vi "Main_001.vi"() -> ()   [LabVIEW 2018]
uses:
  Control/State_01.ctl
  <vilib>/vision/Image Controls.llb/IMAQ Image.ctl
  <vilib>/Utility/miscctls.llb/LVRectTypeDef.ctl
  <vilib>/Utility/miscctls.llb/LVPointTypeDef.ctl
  <vilib>/Utility/file.llb/Write Delimited Spreadsheet (string).vi
  <vilib>/vision/NI_Vision_Development_Module.lvlib
panel:
  out "OCR":bool
  out "Batch":bool
  in  "BatchCycle_Control":u32
  out "BatchCycle":u32
  out "stripped path":path
  in  "Type of Symmetry 4":u32(ring) items=["Horizontal", "Vertical", "Central", "1st Diagonal", "2nd Diagonal"]
  in  "Type of Symmetry":u32(ring)=1 items=["Horizontal", "Vertical", "Central", "1st Diagonal", "2nd Diagonal"]
  in  "Type of Symmetry 3":u32(ring)=1 items=["Horizontal", "Vertical", "Central", "1st Diagonal", "2nd Diagonal"]
  in  "Type of Symmetry 2":u32(ring)=2 items=["Horizontal", "Vertical", "Central", "1st Diagonal", "2nd Diagonal"]
  in  "TrainFile Path":path=path "D:/Life/20191001_Accordance/Project/EPISIL/20200806-Camera/LabVIEW_Test/OCR"
  in  "error in (no error)":errorcluster
  out "error out":errorcluster
  in  "Button_Batch":bool
  in  "Button_EXIT":bool
  out "Result_04":string
  out "Result_03":string
  out "Result_02":string
  out "Result_01":string
  in  "Button_OCR":bool
  in  "Button_ROI":bool
  in  "Erode_04":i32
  in  "Dilate_04":i32
  in  "Y+H_04":i32=990
  in  "X_04":i32=1330
  in  "Y_04":i32=1050
  in  "X+W_04":i32=1390
  out "Show_04":T1(plugin-control)
  in  "Erode_03":i32
  in  "Dilate_03":i32
  in  "Y+H_03":i32=890
  in  "X_03":i32=1380
  in  "Y_03":i32=960
  in  "X+W_03":i32=1450
  out "Show_03":T1(plugin-control)
  in  "Erode_02":i32
  in  "Dilate_02":i32
  in  "Y+H_02":i32=1000
  in  "X_02":i32=650
  in  "Y_02":i32=910
  in  "X+W_02":i32=870
  out "Show_02":T1(plugin-control)
  in  "Binary Value":i32
  in  "Erode_01":i32
  in  "Dilate_01":i32
  in  "Y+H_01":i32=400
  in  "X_01":i32=685
  in  "Y_01":i32=300
  in  "X+W_01":i32=885
  in  "ImagePath":path=path "D:/Life/20191001_Accordance/Project/EPISIL/20200806-Camera/20200716/getimg_003.bmp"
  out "Show_01":T1(plugin-control)
  # "X"
  # "Y"
  # "X+W"
  # "Y+H"
  # "Dilate"
  # "Erode"
  # "X"
  # "Y"
  # "X+W"
  # "Y+H"
  # "Dilate"
  # "Erode"
  # "X"
  # "Y"
  # "X+W"
  # "Y+H"
  # "Dilate"
  # "Erode"
  # "X"
  # "Y"
  # "X+W"
  # "Y+H"
  # "Dilate"
  # "Erode"
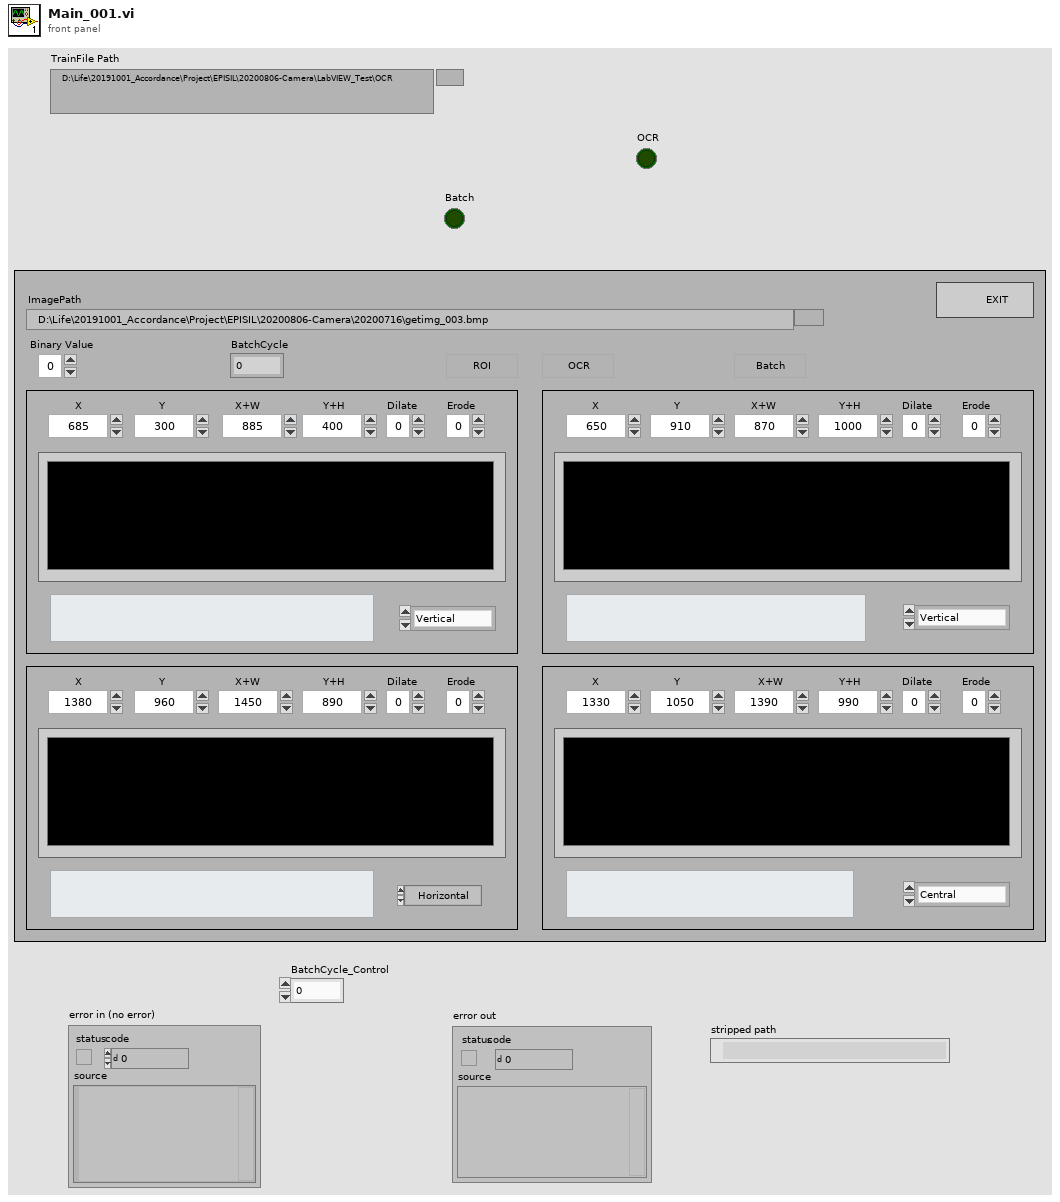
[diagram p1: front panel]
types:
  T1 = typedef "IMAQ Image.ctl" = refnum<image>
  T2 = typedef "State_01.ctl" = enum16{"Inital", "Disable", "Idle", "Display", "BatchCompare", "ROI_01", "ROI_02", "ROI_03", "ROI_04", "OCR", "SaveResult", "EXIT"}
  T3 = typedef "IMAQ OCR Session.ctl" = refnum<k1>
  T4 = typedef "LVPointTypeDef.ctl" = cluster{"Horizontal":i16, "Vertical":i16}
  T5 = typedef "LVRectTypeDef.ctl" = cluster{"Left":i16, "Top":i16, "Right":i16, "Bottom":i16}
  T6 = typedef "IMAQ Rectangle" = cluster{"Left":i32, "Top":i32, "Right":i32, "Bottom":i32, "Rotation":dbl}
  T7 = typedef "Image Type" = u32
  T8 = typedef "ROI Descriptor" = cluster{"Global Rectangle":i32[], "Contours":cluster{"ID":enum32{"External", "Internal"}, "Type":u32, "Coordinates":i32[]}[]}
  T9 = cluster{"Global Rectangle":i32[], "Contours":cluster{"ID":enum32{"External", "Internal"}, "Type":u32, "Coordinates":i32[]}[]}
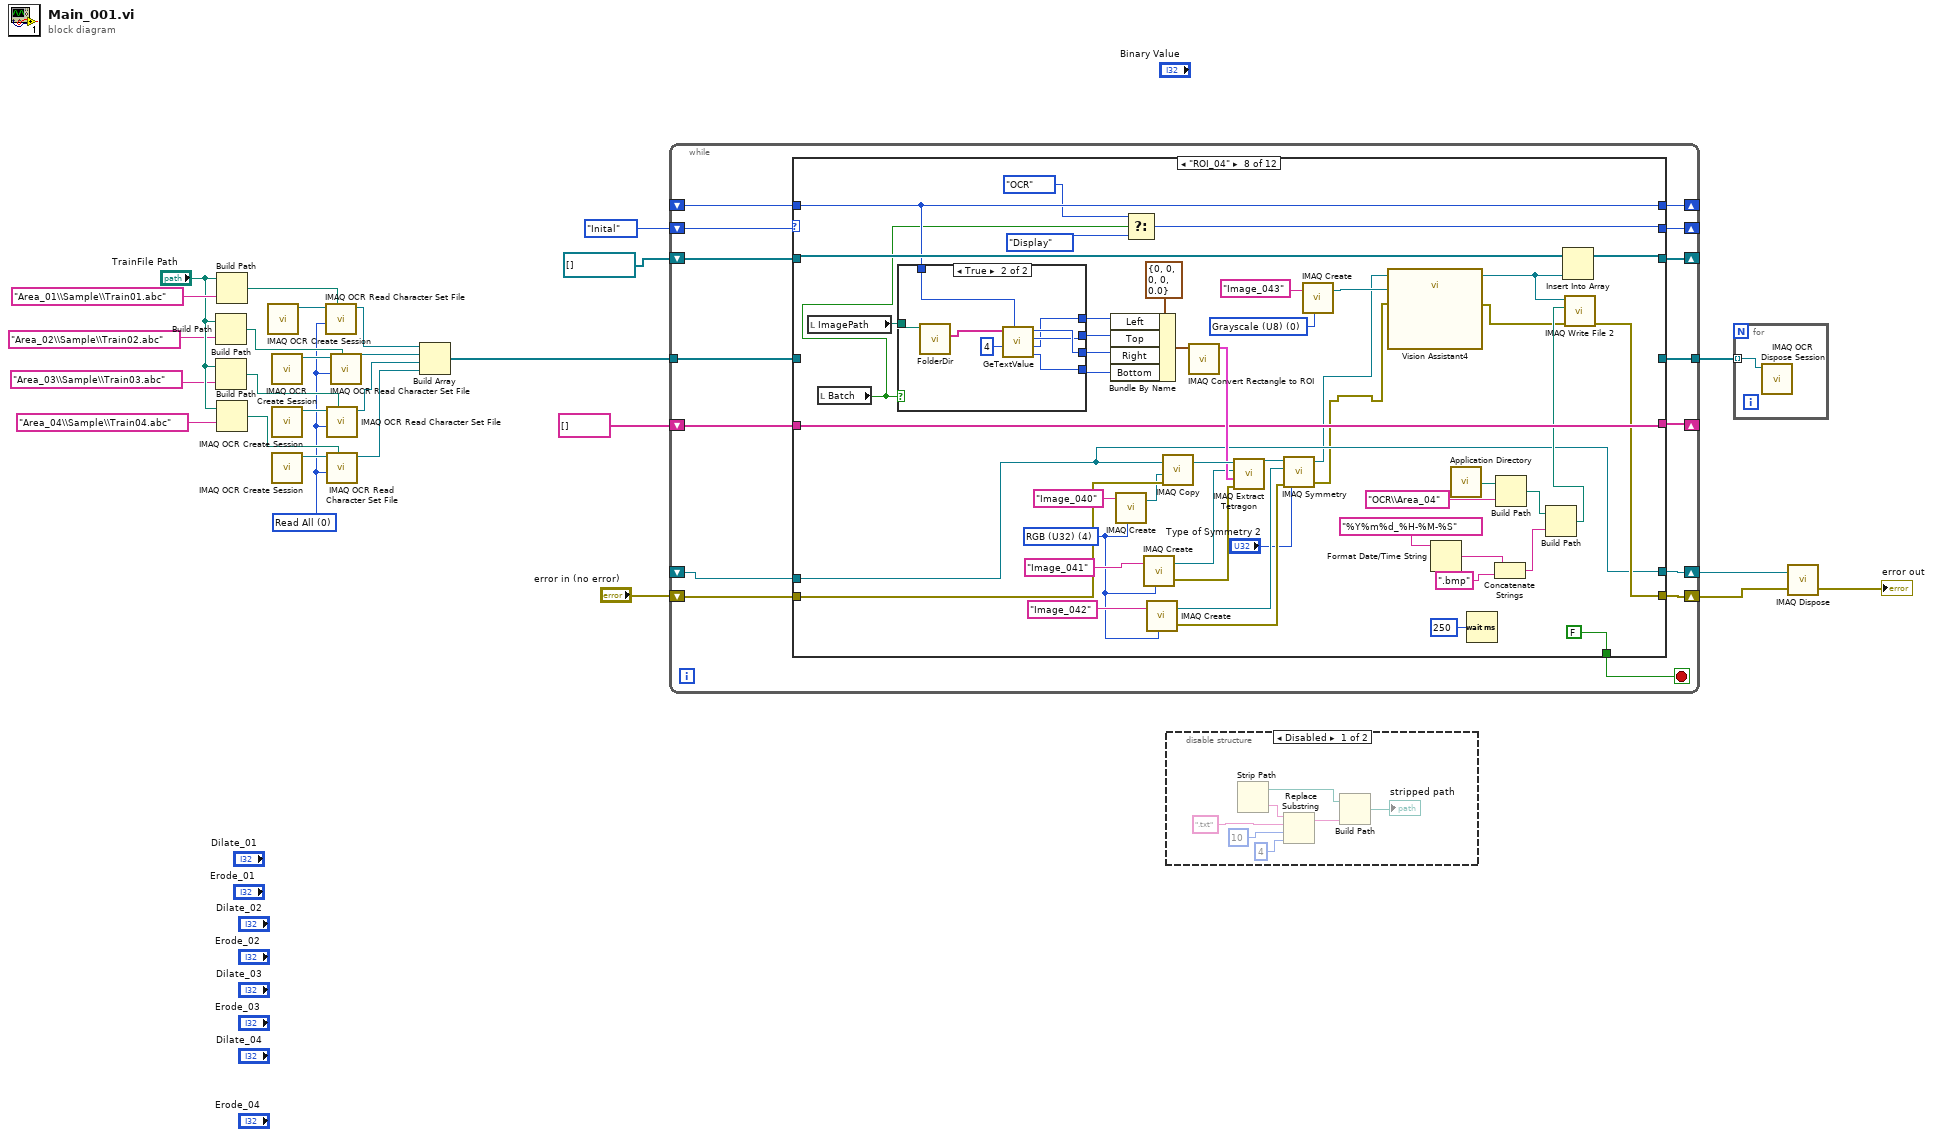
[diagram p0: block diagram]
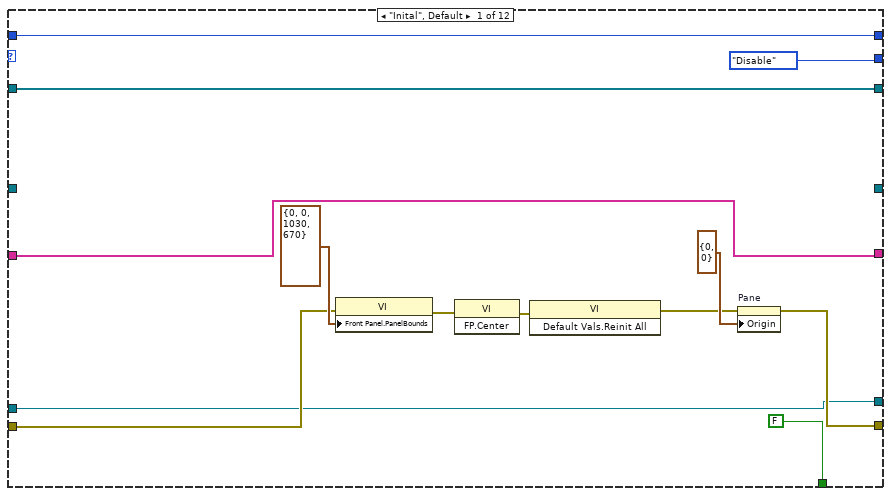
[diagram p3: hidden frame]
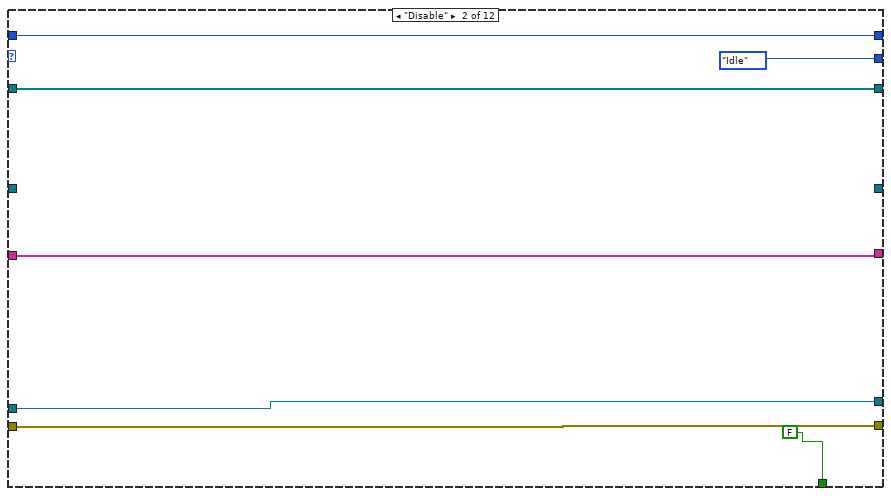
[diagram p4: hidden frame]
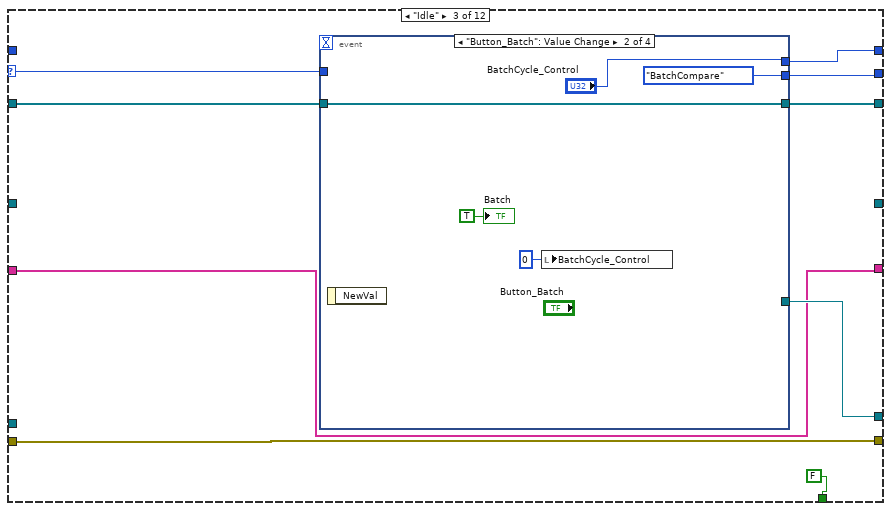
[diagram p5: hidden frame]
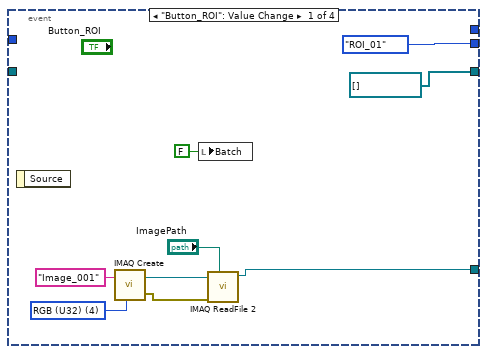
[diagram p6: hidden frame]
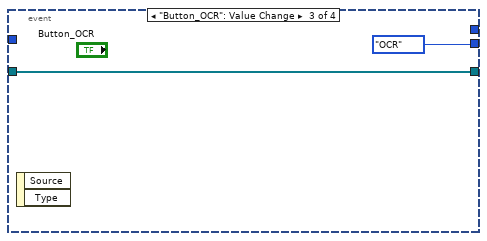
[diagram p7: hidden frame]
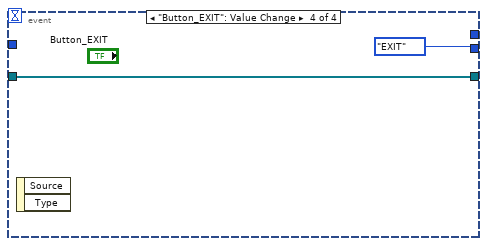
[diagram p8: hidden frame]
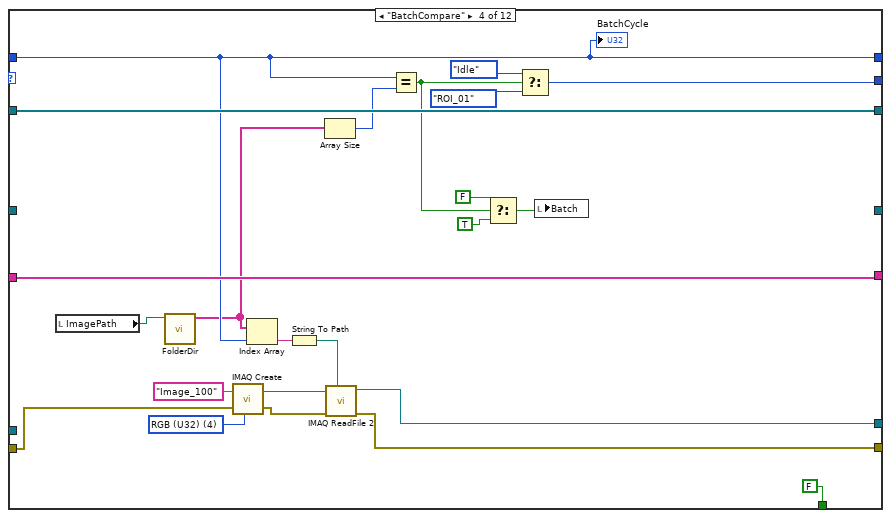
[diagram p9: hidden frame]
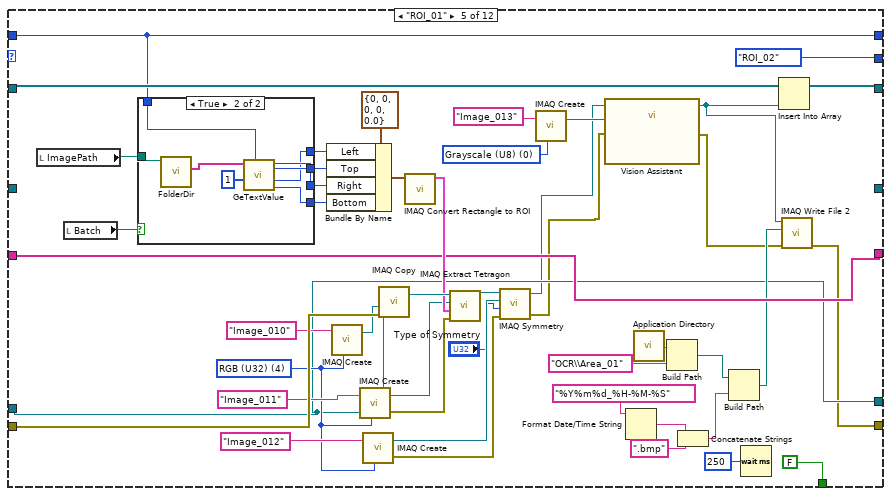
[diagram p10: hidden frame]
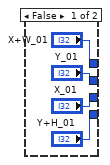
[diagram p11: hidden frame]
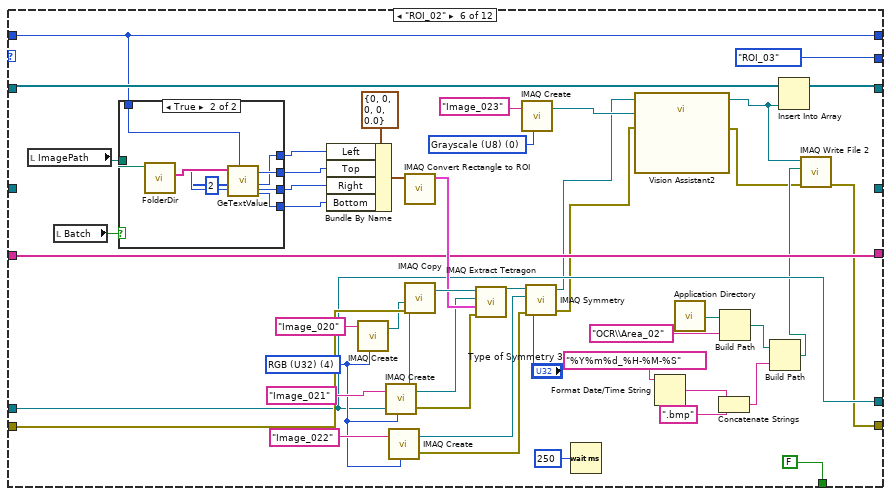
[diagram p12: hidden frame]
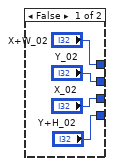
[diagram p13: hidden frame]
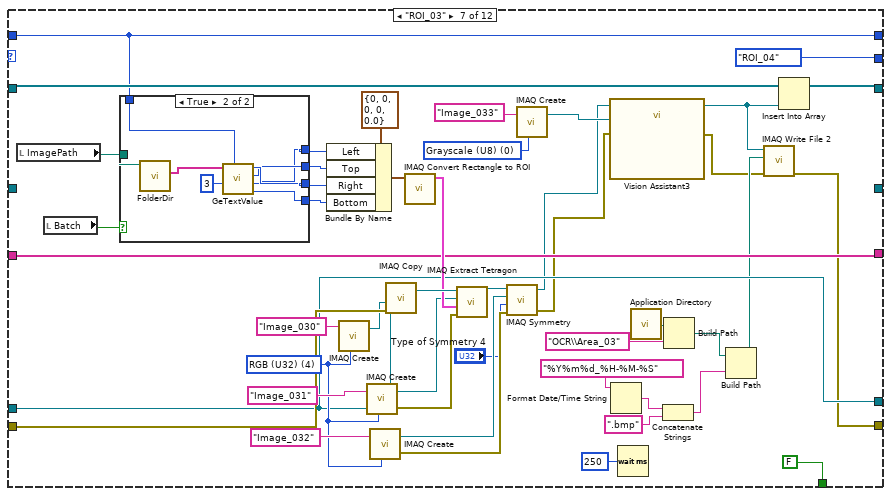
[diagram p14: hidden frame]
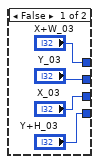
[diagram p15: hidden frame]
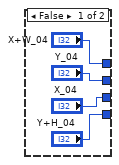
[diagram p16: hidden frame]
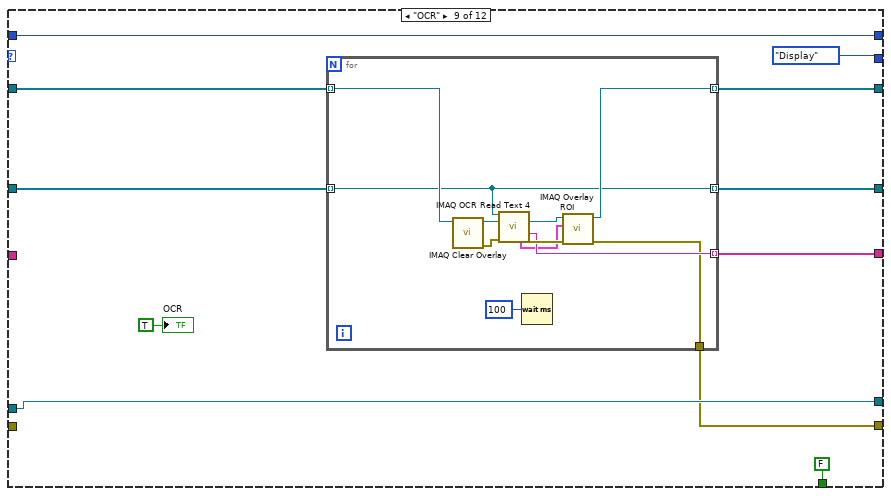
[diagram p17: hidden frame]
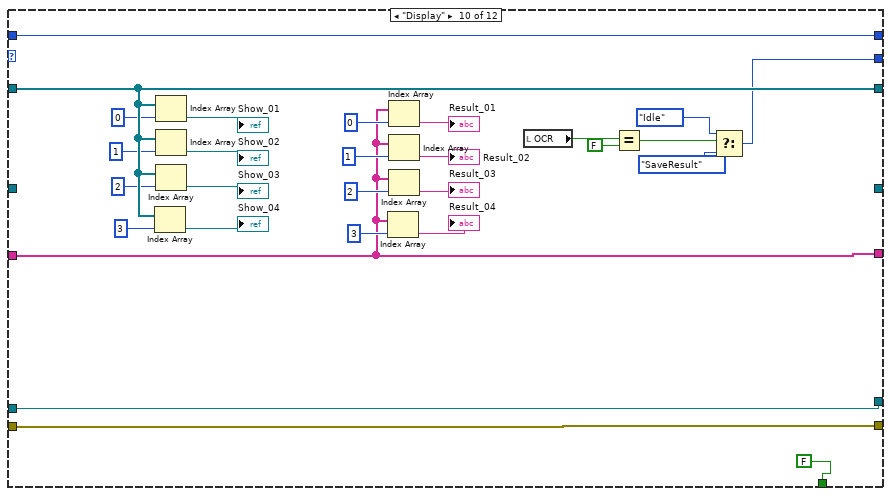
[diagram p18: hidden frame]
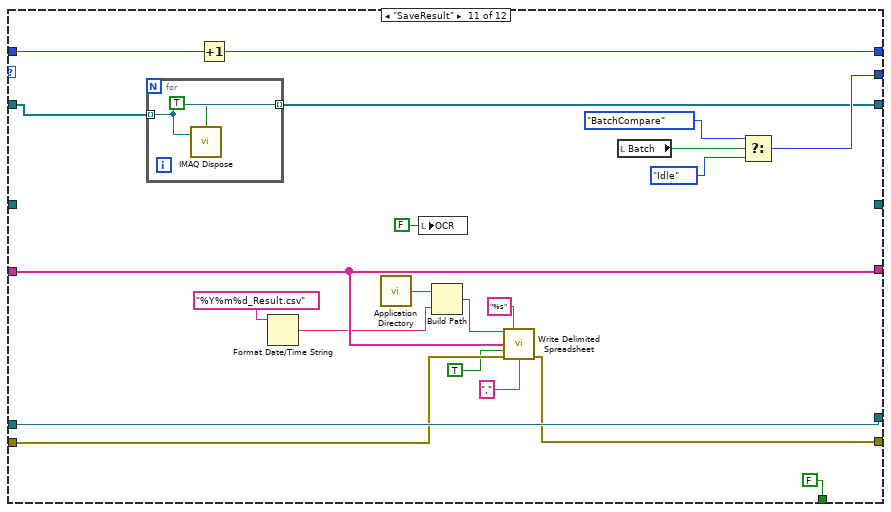
[diagram p19: hidden frame]
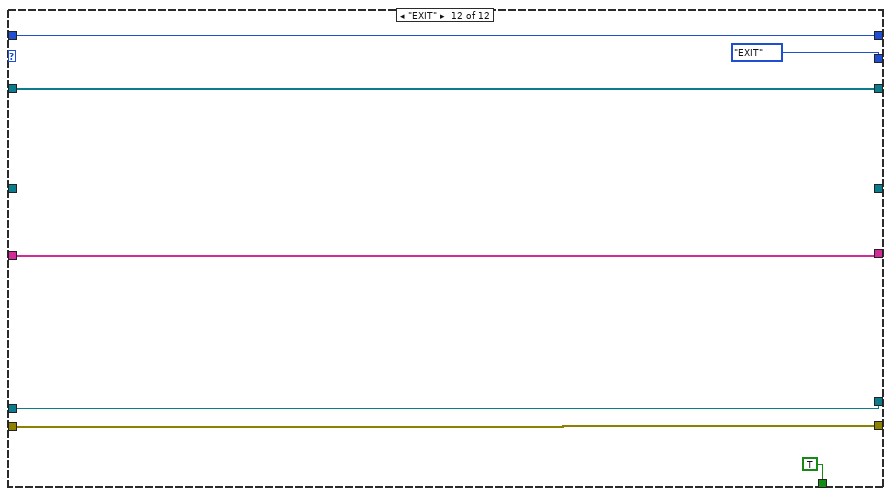
[diagram p20: hidden frame]
diagram:
  w7 = 0 items=["Read All", "Read Character Set Only", "Read Properties Only"] ("Read Options")
  n1 = Build Path(base path="TrainFile Path", name or relative path="Area_02\\Sample\\Train02.abc") -> (appended path=w12:path)
  n2 = Build Path(base path="TrainFile Path", name or relative path="Area_03\\Sample\\Train03.abc") -> (appended path=w11:path)
  n3 = Build Path(base path="TrainFile Path", name or relative path="Area_01\\Sample\\Train01.abc") -> (appended path=w15:path)
  n4 = Build Path(base path="TrainFile Path", name or relative path="Area_04\\Sample\\Train04.abc") -> (appended path=w10:path)
  n5 = call "IMAQ OCR Create Session"() -> ("IMAQ OCR Session"=w14:T3)  [unwired: 10 in, 1 out]
  n6 = call "IMAQ OCR Create Session"() -> ("IMAQ OCR Session"=w13:T3)  [unwired: 10 in, 1 out]
  n7 = call "IMAQ OCR Create Session"() -> ("IMAQ OCR Session"=w8:T3)  [unwired: 10 in, 1 out]
  n8 = call "IMAQ OCR Create Session"() -> ("IMAQ OCR Session"=w9:T3)  [unwired: 10 in, 1 out]
  n9 = call "IMAQ OCR Read Character Set File"("File Path"=w15, "Read Options"=w7, "IMAQ OCR Session"=w14) -> ("IMAQ OCR Session (dup)"=w6:T3)  [unwired: 6 in, 2 out]
  n10 = call "IMAQ OCR Read Character Set File"("File Path"=w11, "Read Options"=w7, "IMAQ OCR Session"=w8) -> ("IMAQ OCR Session (dup)"=w4:T3)  [unwired: 6 in, 2 out]
  n11 = call "IMAQ OCR Read Character Set File"("File Path"=w10, "Read Options"=w7, "IMAQ OCR Session"=w9) -> ("IMAQ OCR Session (dup)"=w3:T3)  [unwired: 6 in, 2 out]
  n12 = call "IMAQ OCR Read Character Set File"("File Path"=w12, "Read Options"=w7, "IMAQ OCR Session"=w13) -> ("IMAQ OCR Session (dup)"=w5:T3)  [unwired: 6 in, 2 out]
  n13 = Build Array(w6, w5, w4, w3) -> (w2:T3[])
  n14 = while {
    shift-right: [w41] -> w27
    shift-left: "error in (no error)" -> [w35]
    shift-right: [w39] -> _
    shift-left: T1[] [] -> [w42]
    shift-right: [w38] -> w25
    shift-left: _ -> [w34]
    shift-right: [w37] -> _
    shift-left: string[] [] -> [w36]
    shift-right: [w32] -> _
    shift-left: State_01."Inital" ("State_01") -> [w33]
    shift-right: [w31] -> _
    shift-left: _ -> [w30]
    tunnel: w2 -> [w29]
    tunnel: [w28] -> w1
    stop <- w40 stop-if-true
    n15 = case shown="\"ROI_04\"" w33 {
      selector: w33 -> [_ _ w69 _ _ _ _ _ _ _ _ _]
      tunnel: w42 -> [w47 w61 w70 w110 w144 w206 w264 w324 w356 w390 w398 w425]
      tunnel: w35 -> [w53 w60 w67 w92 w155 w213 w271 w331 _ w395 w407 w426]
      tunnel: [w49 w60 w67 w91 w115 w173 w231 w290 w349 w395 w406 w426] -> w41
      tunnel: [FALSE FALSE FALSE FALSE FALSE FALSE FALSE FALSE FALSE FALSE FALSE TRUE] -> w40
      tunnel: [w47 w61 w68 w110 w143 w205 w263 w323 w355 w390 w397 w425] -> w39
      tunnel: [w45 w58 w66 w93 w117 w192 w251 w289 w353 w376 w417 w422] -> w38
      tunnel: [w46 w59 w65 w112 w131 w193 w252 w311 w354 w381 w401 w423] -> w37
      tunnel: w36 -> [w46 w59 w65 w112 w131 w193 w252 w311 _ w381 w401 w423]
      tunnel: w34 -> [w45 w58 _ _ w117 w192 w251 w289 w353 w376 w417 w422]
      tunnel: [State_01."Disable" ("State_01") State_01."Idle" ("State_01") w64 w106 State_01."ROI_02" ("State_01") State_01."ROI_03" ("State_01") State_01."ROI_04" ("State_01") w292 State_01."Display" ("State_01") w371 w410 State_01."EXIT" ("State_01")] -> w32
      tunnel: [w43 w56 w63 w96 w118 w175 w237 w300 w351 w375 w414 w420] -> w31
      tunnel: w30 -> [w43 w56 _ w96 w118 w175 w237 w300 w351 w375 w415 w420]
      tunnel: w29 -> [_ _ _ _ _ _ _ _ w348 _ _ _]
      tunnel: [_ _ _ _ _ _ _ _ w347 _ _ _] -> w28
      frame "Inital", Default {
        n16 = property class="VI"(error in=w53, "Front Panel.PanelBounds"=T5 {"Left"=0, "Top"=0, "Right"=1030, "Bottom"=670} ("Front Panel Window:Panel Bounds")) -> (error out=w52:errorcluster)  [unwired: 1 in, 1 out]
        n17 = invoke class="VI" method="FP.Center"(error in=w52) -> (error out=w51:errorcluster)  [unwired: 2 in, 2 out]
        n18 = invoke class="VI" method="Default Vals.Reinit All"(error in=w51) -> (error out=w50:errorcluster)  [unwired: 2 in, 2 out]
        n19 = property on="Pane" class="Pane"(error in=w50, "Origin"=T4 {"Horizontal"=0, "Vertical"=0}) -> (error out=w49:errorcluster)  [unwired: 1 in, 1 out]
      }
      frame "Disable" {
      }
      frame "Idle" {
        n20 = event shown="[1] \"Button_Batch\": Value Change" {
          selector: _ -> [_ _ _ _]
          dyn-events: _ -> [_ _ _ _]
          timeout: _ -> [_ _ _ _]
          tunnel: w70 -> [_ w85 w87 w89]
          tunnel: w69 -> [_ _ _ _]
          tunnel: [State_01."ROI_01" ("State_01") State_01."BatchCompare" ("State_01") State_01."OCR" ("State_01") State_01."EXIT" ("State_01")] -> w64
          tunnel: [T1[] [] w85 w87 w89] -> w68
          tunnel: [w77 _ _ _] -> w66
          tunnel: [_ "BatchCycle_Control" _ _] -> w63
          event "Button_ROI": Value Change {
            w75 = T7 4 items=["Grayscale (U8)", "Grayscale (I16)", "Grayscale (SGL)", "Complex (CSG)", "RGB (U32)", "HSL (U32)", "RGB (U64)", "Grayscale (U16)"] ("Image Type")
            n21 = event-data() -> ()  [unwired: 1 in, 1 out]
            n22 = call "IMAQ Create"("Image Name"="Image_001", "Image Type"=w75) -> ("New Image"=w74:T1, "error out"=w73:errorcluster)  [unwired: 3 in]
            n23 = local write "Batch"(FALSE ("Batch")) -> ()
            n24 = call "IMAQ ReadFile 2"("File Path"="ImagePath", "error in (no error)"=w73, "Image"=w74) -> ("Image Out"=w77:T1)  [unwired: 4 in, 4 out]
          }
          event "Button_Batch": Value Change {
            n25 = event-data() -> ()  [unwired: 1 in, 1 out]
            n26 = local write "BatchCycle_Control"(u32 0 ("BatchCycle_Control")) -> ()
            "Batch" <- TRUE ("Batch")
          }
          event "Button_OCR": Value Change {
            n27 = event-data() -> ()  [unwired: 1 in, 2 out]
          }
          event "Button_EXIT": Value Change {
            n28 = event-data() -> ()  [unwired: 1 in, 2 out]
          }
        }
      }
      frame "BatchCompare" {
        w100 = T7 4 items=["Grayscale (U8)", "Grayscale (I16)", "Grayscale (SGL)", "Complex (CSG)", "RGB (U32)", "HSL (U32)", "RGB (U64)", "Grayscale (U16)"] ("Image Type")
        n29 = local read "ImagePath"() -> (w99:path)
        n30 = call "FolderDir.vi"("ImagePath"=w99) -> ("ArrayImage"=w90:string[])  [unwired: 8 in, 2 out]
        n31 = call "IMAQ Create"("Image Name"="Image_100", "Image Type"=w100, "error in (no error)"=w92) -> ("New Image"=w97:T1, "error out"=w101:errorcluster)  [unwired: 2 in]
        n32 = Index Array(array=w90, index=w96) -> (element=w95:string)
        n33 = String To Path(string=w95) -> (path=w94:path)
        n34 = Array Size(array=w90) -> (size(s)=w109:i32)
        n35 = call "IMAQ ReadFile 2"("File Path"=w94, "error in (no error)"=w101, "Image"=w97) -> ("error out"=w91:errorcluster, "Image Out"=w93:T1)  [unwired: 4 in, 3 out]
        n36 = Equal?(x=w96, y=w109) -> (x = y?=w105:bool)
        n37 = Select(t=FALSE, s=w105, f=TRUE) -> (s? t:f=w102:bool)
        n38 = Select(t=State_01."Idle" ("State_01"), s=w105, f=State_01."ROI_01" ("State_01")) -> (s? t:f=w106:T2)
        n39 = local write "Batch"(w102) -> ()
        "BatchCycle" <- w96
      }
      frame "ROI_01" {
        w138 = T7 0 items=["Grayscale (U8)", "Grayscale (I16)", "Grayscale (SGL)", "Complex (CSG)", "RGB (U32)", "HSL (U32)", "RGB (U64)", "Grayscale (U16)"] ("Image Type")
        w141 = T7 4 items=["Grayscale (U8)", "Grayscale (I16)", "Grayscale (SGL)", "Complex (CSG)", "RGB (U32)", "HSL (U32)", "RGB (U64)", "Grayscale (U16)"] ("Image Type")
        n40 = local read "ImagePath"() -> (w119:path)
        n41 = local read "Batch"() -> (w120:bool)
        n42 = case shown="True" w120 {
          tunnel: ["X+W_01" w165] -> w152
          tunnel: ["Y_01" w166] -> w151
          tunnel: ["X_01" w167] -> w150
          tunnel: ["Y+H_01" w164] -> w149
          tunnel: w119 -> [_ w170]
          tunnel: w118 -> [_ w168]
          frame False {
          }
          frame True {
            n43 = call "FolderDir.vi"("ImagePath"=w170) -> ("ArrayTxt"=w169:string[])  [unwired: 8 in, 2 out]
            n44 = call "GeTextValue.vi"("index"=w168, "Area"=1, "ArrayTxt"=w169) -> ("Y+H"=w164:i32, "X+W"=w165:i32, "Y"=w166:i32, "X"=w167:i32)  [unwired: 4 in, 1 out]
          }
        }
        n45 = Bundle By Name(cluster=T6 {"Left"=0, "Top"=0, "Right"=0, "Bottom"=0, "Rotation"=0.0} ("Rectangle"), "Left"=w152, "Top"=w151, "Right"=w150, "Bottom"=w149) -> (w156:T6)
        n46 = call "IMAQ Create"("Image Name"="Image_010", "Image Type"=w141) -> ("New Image"=w153:T1)  [unwired: 3 in, 1 out]
        n47 = call "IMAQ Create"("Image Name"="Image_011", "Image Type"=w141) -> ("New Image"=w145:T1, "error out"=w135:errorcluster)  [unwired: 3 in]
        n48 = call "IMAQ Create"("Image Name"="Image_012", "Image Type"=w141) -> ("New Image"=w140:T1, "error out"=w134:errorcluster)  [unwired: 3 in]
        n49 = call "IMAQ Copy"("error in (no error)"=w155, "Image Dst"=w153, "Image Src"=w117) -> ("Image Dst Out"=w148:T1)  [unwired: 3 in, 1 out]
        n50 = call "IMAQ Convert Rectangle to ROI"("Rectangle"=w156) -> ("ROI Descriptor"=w147:T8)  [unwired: 8 in, 1 out]
        n51 = call-poly "IMAQ Extract Tetragon"("error in (no error)"=w135, "ROI Descriptor"=w147, "Image Dst"=w145, "Image Src"=w148) -> ("Image Dst Out"=w139:T1)  [unwired: 6 in, 1 out]
        n52 = call "IMAQ Symmetry"("error in (no error)"=w134, "Type of Symmetry"="Type of Symmetry", "Image Dst"=w140, "Image Src"=w139) -> ("error out"=w114:errorcluster, "Image Dst Out"=w113:T1)  [unwired: 1 in]
        n53 = call "IMAQ Create"("Image Name"="Image_013", "Image Type"=w138) -> ("New Image"=w136:T1)  [unwired: 3 in, 1 out]
        n54 = call "Vision Assistant"("Image In"=w113, "Image Dst"=w136, "error in"=w114) -> ("Image Out"=w132:T1, "error out"=w116:errorcluster)  [unwired: 23 in]
        n55 = Format Date/Time String(time format string (%c)="%Y%m%d_%H-%M-%S") -> (date/time string=w126:string)  [unwired: 2 in]
        n56 = call <vilib>:"Application Directory.vi"() -> ("Application Directory"=w130:path)
        n57 = Build Path(base path=w130, name or relative path="OCR\\Area_01") -> (appended path=w127:path)
        n58 = Concatenate Strings(w126, ".bmp" ("string")) -> (w123:string)
        n59 = Build Path(base path=w127, name or relative path=w123) -> (appended path=w122:path)
        n60 = Wait (ms)(milliseconds to wait=u32 250) -> ()  [unwired: 1 out]
        n61 = Insert Into Array(array=w144, new element=w132) -> (w143:T1[])  [unwired: 1 in]
        n62 = call-poly "IMAQ Write File 2"("error in (no error)"=w116, "File Path"=w122, "Image"=w132) -> ("error out"=w115:errorcluster)  [unwired: 7 in, 1 out]
      }
      frame "ROI_02" {
        w200 = T7 0 items=["Grayscale (U8)", "Grayscale (I16)", "Grayscale (SGL)", "Complex (CSG)", "RGB (U32)", "HSL (U32)", "RGB (U64)", "Grayscale (U16)"] ("Image Type")
        w203 = T7 4 items=["Grayscale (U8)", "Grayscale (I16)", "Grayscale (SGL)", "Complex (CSG)", "RGB (U32)", "HSL (U32)", "RGB (U64)", "Grayscale (U16)"] ("Image Type")
        n63 = local read "ImagePath"() -> (w180:path)
        n64 = local read "Batch"() -> (w181:bool)
        n65 = case shown="True" w181 {
          tunnel: ["X+W_02" w223] -> w179
          tunnel: ["Y_02" w224] -> w178
          tunnel: ["X_02" w225] -> w177
          tunnel: ["Y+H_02" w222] -> w176
          tunnel: w180 -> [_ w228]
          tunnel: w175 -> [_ w226]
          frame False {
          }
          frame True {
            n66 = call "FolderDir.vi"("ImagePath"=w228) -> ("ArrayTxt"=w227:string[])  [unwired: 8 in, 2 out]
            n67 = call "GeTextValue.vi"("index"=w226, "Area"=2, "ArrayTxt"=w227) -> ("Y+H"=w222:i32, "X+W"=w223:i32, "Y"=w224:i32, "X"=w225:i32)  [unwired: 4 in, 1 out]
          }
        }
        n68 = Bundle By Name(cluster=T6 {"Left"=0, "Top"=0, "Right"=0, "Bottom"=0, "Rotation"=0.0} ("Rectangle"), "Left"=w179, "Top"=w178, "Right"=w177, "Bottom"=w176) -> (w214:T6)
        n69 = call "IMAQ Create"("Image Name"="Image_020", "Image Type"=w203) -> ("New Image"=w211:T1)  [unwired: 3 in, 1 out]
        n70 = call "IMAQ Create"("Image Name"="Image_021", "Image Type"=w203) -> ("New Image"=w207:T1, "error out"=w197:errorcluster)  [unwired: 3 in]
        n71 = call "IMAQ Create"("Image Name"="Image_022", "Image Type"=w203) -> ("New Image"=w202:T1, "error out"=w196:errorcluster)  [unwired: 3 in]
        n72 = call "IMAQ Convert Rectangle to ROI"("Rectangle"=w214) -> ("ROI Descriptor"=w209:T8)  [unwired: 8 in, 1 out]
        n73 = call "IMAQ Copy"("error in (no error)"=w213, "Image Dst"=w211, "Image Src"=w192) -> ("Image Dst Out"=w210:T1)  [unwired: 3 in, 1 out]
        n74 = call-poly "IMAQ Extract Tetragon"("error in (no error)"=w197, "ROI Descriptor"=w209, "Image Dst"=w207, "Image Src"=w210) -> ("Image Dst Out"=w201:T1)  [unwired: 6 in, 1 out]
        n75 = call "IMAQ Create"("Image Name"="Image_023", "Image Type"=w200) -> ("New Image"=w198:T1)  [unwired: 3 in, 1 out]
        n76 = call "IMAQ Symmetry"("error in (no error)"=w196, "Type of Symmetry"="Type of Symmetry 3", "Image Dst"=w202, "Image Src"=w201) -> ("error out"=w172:errorcluster, "Image Dst Out"=w171:T1)  [unwired: 1 in]
        n77 = Wait (ms)(milliseconds to wait=u32 250) -> ()  [unwired: 1 out]
        n78 = call "Vision Assistant2"("Image In"=w171, "Image Dst"=w198, "error in"=w172) -> ("Image Out"=w194:T1, "error out"=w174:errorcluster)  [unwired: 23 in]
        n79 = Format Date/Time String(time format string (%c)="%Y%m%d_%H-%M-%S") -> (date/time string=w186:string)  [unwired: 2 in]
        n80 = call <vilib>:"Application Directory.vi"() -> ("Application Directory"=w190:path)
        n81 = Concatenate Strings(w186, ".bmp" ("string")) -> (w184:string)
        n82 = Build Path(base path=w190, name or relative path="OCR\\Area_02") -> (appended path=w187:path)
        n83 = Build Path(base path=w187, name or relative path=w184) -> (appended path=w183:path)
        n84 = Insert Into Array(array=w206, new element=w194) -> (w205:T1[])  [unwired: 1 in]
        n85 = call-poly "IMAQ Write File 2"("error in (no error)"=w174, "File Path"=w183, "Image"=w194) -> ("error out"=w173:errorcluster)  [unwired: 7 in, 1 out]
      }
      frame "ROI_03" {
        w258 = T7 0 items=["Grayscale (U8)", "Grayscale (I16)", "Grayscale (SGL)", "Complex (CSG)", "RGB (U32)", "HSL (U32)", "RGB (U64)", "Grayscale (U16)"] ("Image Type")
        w261 = T7 4 items=["Grayscale (U8)", "Grayscale (I16)", "Grayscale (SGL)", "Complex (CSG)", "RGB (U32)", "HSL (U32)", "RGB (U64)", "Grayscale (U16)"] ("Image Type")
        n86 = local read "ImagePath"() -> (w238:path)
        n87 = local read "Batch"() -> (w239:bool)
        n88 = case shown="True" w239 {
          tunnel: ["X+W_03" w281] -> w236
          tunnel: ["Y_03" w282] -> w235
          tunnel: ["X_03" w283] -> w234
          tunnel: ["Y+H_03" w280] -> w233
          tunnel: w238 -> [_ w286]
          tunnel: w237 -> [_ w284]
          frame False {
          }
          frame True {
            n89 = call "FolderDir.vi"("ImagePath"=w286) -> ("ArrayTxt"=w285:string[])  [unwired: 8 in, 2 out]
            n90 = call "GeTextValue.vi"("index"=w284, "Area"=3, "ArrayTxt"=w285) -> ("Y+H"=w280:i32, "X+W"=w281:i32, "Y"=w282:i32, "X"=w283:i32)  [unwired: 4 in, 1 out]
          }
        }
        n91 = Bundle By Name(cluster=T6 {"Left"=0, "Top"=0, "Right"=0, "Bottom"=0, "Rotation"=0.0} ("Rectangle"), "Left"=w236, "Top"=w235, "Right"=w234, "Bottom"=w233) -> (w272:T6)
        n92 = call "IMAQ Create"("Image Name"="Image_030", "Image Type"=w261) -> ("New Image"=w269:T1)  [unwired: 3 in, 1 out]
        n93 = call "IMAQ Create"("Image Name"="Image_031", "Image Type"=w261) -> ("New Image"=w265:T1, "error out"=w255:errorcluster)  [unwired: 3 in]
        n94 = call "IMAQ Create"("Image Name"="Image_032", "Image Type"=w261) -> ("New Image"=w260:T1, "error out"=w254:errorcluster)  [unwired: 3 in]
        n95 = call "IMAQ Copy"("error in (no error)"=w271, "Image Dst"=w269, "Image Src"=w251) -> ("Image Dst Out"=w268:T1)  [unwired: 3 in, 1 out]
        n96 = call "IMAQ Convert Rectangle to ROI"("Rectangle"=w272) -> ("ROI Descriptor"=w267:T8)  [unwired: 8 in, 1 out]
        n97 = call-poly "IMAQ Extract Tetragon"("error in (no error)"=w255, "ROI Descriptor"=w267, "Image Dst"=w265, "Image Src"=w268) -> ("Image Dst Out"=w259:T1)  [unwired: 6 in, 1 out]
        n98 = call "IMAQ Symmetry"("error in (no error)"=w254, "Type of Symmetry"="Type of Symmetry 4", "Image Dst"=w260, "Image Src"=w259) -> ("error out"=w230:errorcluster, "Image Dst Out"=w229:T1)  [unwired: 1 in]
        n99 = call "IMAQ Create"("Image Name"="Image_033", "Image Type"=w258) -> ("New Image"=w256:T1)  [unwired: 3 in, 1 out]
        n100 = call "Vision Assistant3"("Image In"=w229, "Image Dst"=w256, "error in"=w230) -> ("Image Out"=w253:T1, "error out"=w232:errorcluster)  [unwired: 23 in]
        n101 = Format Date/Time String(time format string (%c)="%Y%m%d_%H-%M-%S") -> (date/time string=w245:string)  [unwired: 2 in]
        n102 = Wait (ms)(milliseconds to wait=u32 250) -> ()  [unwired: 1 out]
        n103 = call <vilib>:"Application Directory.vi"() -> ("Application Directory"=w249:path)
        n104 = Concatenate Strings(w245, ".bmp" ("string")) -> (w243:string)
        n105 = Build Path(base path=w249, name or relative path="OCR\\Area_03") -> (appended path=w246:path)
        n106 = Build Path(base path=w246, name or relative path=w243) -> (appended path=w242:path)
        n107 = call-poly "IMAQ Write File 2"("error in (no error)"=w232, "File Path"=w242, "Image"=w253) -> ("error out"=w231:errorcluster)  [unwired: 7 in, 1 out]
        n108 = Insert Into Array(array=w264, new element=w253) -> (w263:T1[])  [unwired: 1 in]
      }
      frame "ROI_04" {
        w318 = T7 0 items=["Grayscale (U8)", "Grayscale (I16)", "Grayscale (SGL)", "Complex (CSG)", "RGB (U32)", "HSL (U32)", "RGB (U64)", "Grayscale (U16)"] ("Image Type")
        w321 = T7 4 items=["Grayscale (U8)", "Grayscale (I16)", "Grayscale (SGL)", "Complex (CSG)", "RGB (U32)", "HSL (U32)", "RGB (U64)", "Grayscale (U16)"] ("Image Type")
        n109 = local read "ImagePath"() -> (w301:path)
        n110 = local read "Batch"() -> (w295:bool)
        n111 = case shown="True" w295 {
          tunnel: ["X+W_04" w342] -> w299
          tunnel: ["Y_04" w343] -> w298
          tunnel: ["X_04" w344] -> w297
          tunnel: ["Y+H_04" w341] -> w296
          tunnel: w301 -> [_ w346]
          tunnel: w300 -> [_ w339]
          frame False {
          }
          frame True {
            n112 = call "FolderDir.vi"("ImagePath"=w346) -> ("ArrayTxt"=w345:string[])  [unwired: 8 in, 2 out]
            n113 = call "GeTextValue.vi"("index"=w339, "Area"=4, "ArrayTxt"=w345) -> ("Y+H"=w341:i32, "X+W"=w342:i32, "Y"=w343:i32, "X"=w344:i32)  [unwired: 4 in, 1 out]
          }
        }
        n114 = Bundle By Name(cluster=T6 {"Left"=0, "Top"=0, "Right"=0, "Bottom"=0, "Rotation"=0.0} ("Rectangle"), "Left"=w299, "Top"=w298, "Right"=w297, "Bottom"=w296) -> (w332:T6)
        n115 = call "IMAQ Create"("Image Name"="Image_040", "Image Type"=w321) -> ("New Image"=w329:T1)  [unwired: 3 in, 1 out]
        n116 = Select(t=State_01."OCR" ("State_01"), s=w295, f=State_01."Display" ("State_01")) -> (s? t:f=w292:T2)
        n117 = call "IMAQ Create"("Image Name"="Image_041", "Image Type"=w321) -> ("New Image"=w325:T1, "error out"=w315:errorcluster)  [unwired: 3 in]
        n118 = call "IMAQ Create"("Image Name"="Image_042", "Image Type"=w321) -> ("New Image"=w320:T1, "error out"=w314:errorcluster)  [unwired: 3 in]
        n119 = call "IMAQ Copy"("error in (no error)"=w331, "Image Dst"=w329, "Image Src"=w289) -> ("Image Dst Out"=w328:T1)  [unwired: 3 in, 1 out]
        n120 = call "IMAQ Convert Rectangle to ROI"("Rectangle"=w332) -> ("ROI Descriptor"=w327:T8)  [unwired: 8 in, 1 out]
        n121 = call-poly "IMAQ Extract Tetragon"("error in (no error)"=w315, "ROI Descriptor"=w327, "Image Dst"=w325, "Image Src"=w328) -> ("Image Dst Out"=w319:T1)  [unwired: 6 in, 1 out]
        n122 = call "IMAQ Symmetry"("error in (no error)"=w314, "Type of Symmetry"="Type of Symmetry 2", "Image Dst"=w320, "Image Src"=w319) -> ("error out"=w288:errorcluster, "Image Dst Out"=w287:T1)  [unwired: 1 in]
        n123 = call "IMAQ Create"("Image Name"="Image_043", "Image Type"=w318) -> ("New Image"=w316:T1)  [unwired: 3 in, 1 out]
        n124 = call "Vision Assistant4"("Image In"=w287, "Image Dst"=w316, "error in"=w288) -> ("Image Out"=w312:T1, "error out"=w291:errorcluster)  [unwired: 23 in]
        n125 = Format Date/Time String(time format string (%c)="%Y%m%d_%H-%M-%S") -> (date/time string=w307:string)  [unwired: 2 in]
        n126 = call <vilib>:"Application Directory.vi"() -> ("Application Directory"=w309:path)
        n127 = Wait (ms)(milliseconds to wait=u32 250) -> ()  [unwired: 1 out]
        n128 = Concatenate Strings(w307, ".bmp" ("string")) -> (w306:string)
        n129 = Build Path(base path=w309, name or relative path="OCR\\Area_04") -> (appended path=w308:path)
        n130 = Build Path(base path=w308, name or relative path=w306) -> (appended path=w302:path)
        n131 = Insert Into Array(array=w324, new element=w312) -> (w323:T1[])  [unwired: 1 in]
        n132 = call-poly "IMAQ Write File 2"("error in (no error)"=w291, "File Path"=w302, "Image"=w312) -> ("error out"=w290:errorcluster)  [unwired: 7 in, 1 out]
      }
      frame "OCR" {
        n133 = for {
          tunnel: w356 -> [w362] mode=indexing
          tunnel: [w361] -> w355 mode=indexing
          tunnel: [w365] -> w354 mode=indexing
          tunnel: [w359] -> w349
          tunnel: w348 -> [w358] mode=indexing
          tunnel: [w358] -> w347 mode=indexing
          n134 = call "IMAQ Clear Overlay"("Image"=w362) -> ("error out"=w367:errorcluster, "Image Out"=w368:T1)  [unwired: 9 in]
          n135 = call "IMAQ OCR Read Text 4"("IMAQ OCR Session"=w358, "Image"=w368, "error in (no error)"=w367) -> ("Image (dup)"=w364:T1, "Read String"=w365:string, "ROI Bounding Characters"=w363:T9, "error out"=w366:errorcluster)  [unwired: 6 in, 3 out]
          n136 = Wait (ms)(milliseconds to wait=u32 100) -> ()  [unwired: 1 out]
          n137 = call "IMAQ Overlay ROI"("error in (no error)"=w366, "ROI Descriptor"=w363, "Image"=w364) -> ("error out"=w359:errorcluster, "Image Out"=w361:T1)  [unwired: 7 in]
        }
        "OCR" <- TRUE ("ROI4")
      }
      frame "Display" {
        n138 = Index Array(array=w390, index=3) -> (element=→"Show_04":T1)
        n139 = Index Array(array=w390, index=0) -> (element=→"Show_01":T1)
        n140 = Index Array(array=w390, index=1) -> (element=→"Show_02":T1)
        n141 = Index Array(array=w390, index=2) -> (element=→"Show_03":T1)
        n142 = Index Array(array=w381, index=3) -> (element=→"Result_04":string)
        n143 = Index Array(array=w381, index=0) -> (element=→"Result_01":string)
        n144 = Index Array(array=w381, index=1) -> (element=→"Result_02":string)
        n145 = Index Array(array=w381, index=2) -> (element=→"Result_03":string)
        n146 = local read "OCR"() -> (w370:bool)
        n147 = Equal?(x=w370, y=FALSE) -> (x = y?=w374:bool)
        n148 = Select(t=State_01."Idle" ("State_01"), s=w374, f=State_01."SaveResult" ("State_01")) -> (s? t:f=w371:T2)
      }
      frame "SaveResult" {
        n149 = for {
          tunnel: w398 -> [w419] mode=indexing
          tunnel: [w419] -> w397 mode=indexing
          n150 = call "IMAQ Dispose"("All Images? (No)"=TRUE, "Image"=w419) -> ()  [unwired: 4 in, 1 out]
        }
        n151 = Increment(x=w415) -> (x+1=w414:u32)
        n152 = Format Date/Time String(time format string (%c)="%Y%m%d_Result.csv") -> (date/time string=w399:string)  [unwired: 2 in]
        n153 = call <vilib>:"Application Directory.vi"() -> ("Application Directory"=w404:path)
        n154 = local write "OCR"(FALSE ("OCR")) -> ()
        n155 = Build Path(base path=w404, name or relative path=w399) -> (appended path=w403:path)
        n156 = call-poly <vilib>:"Write Delimited Spreadsheet.vi"("file path (dialog if empty)"=w403, "format (%s)"="%s", "1D data"=w401, "append to file? (new file:F)"=TRUE, "error in (no error)"=w407, "delimiter (\\t)"="," ("delimiter (\\t)")) -> ("error out"=w406:errorcluster)  [unwired: 8 in, 1 out]
        n157 = local read "Batch"() -> (w413:bool)
        n158 = Select(t=State_01."BatchCompare" ("State_01"), s=w413, f=State_01."Idle" ("State_01")) -> (s? t:f=w410:T2)
      }
      frame "EXIT" {
      }
    }
  }
  n159 = disable-structure shown="Disabled" {
    frame Disabled {
      n160 = Strip Path() -> (stripped path=w433:path, name=w432:string)  [unwired: 1 in]
      n161 = Replace Substring(2:4 ("length (len. of substring)"), 3:10 ("offset (0)"), 4:".txt" ("substring (\"\")"), 5:w432) -> (1:w430:string)  [unwired: 1 out]
      n162 = Build Path(base path=w433, name or relative path=w430) -> (appended path=→"stripped path":path)
    }
    frame Enabled {
    }
  }
  n163 = for {
    tunnel: w1 -> [w434] mode=indexing
    n164 = call "IMAQ OCR Dispose Session"("IMAQ OCR Session"=w434) -> ()  [unwired: 10 in, 1 out]
  }
  n165 = call "IMAQ Dispose"("Image"=w25, "error in (no error)"=w27) -> ("error out"=→"error out":errorcluster)  [unwired: 4 in]
